vi "user_events_practice.vi"() -> ()   [LabVIEW 2020]
panel:
  out "all upper case string":string
  in  "Change to Upper":cluster{"string":string}={"string"="exaMple"}
  in  "stop":bool
  out "error out":errorcluster
  out "Type":u32
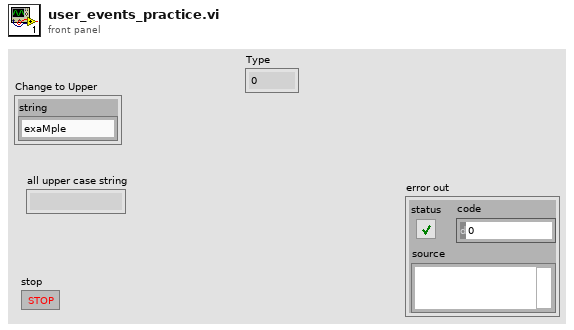
[diagram p1: front panel]
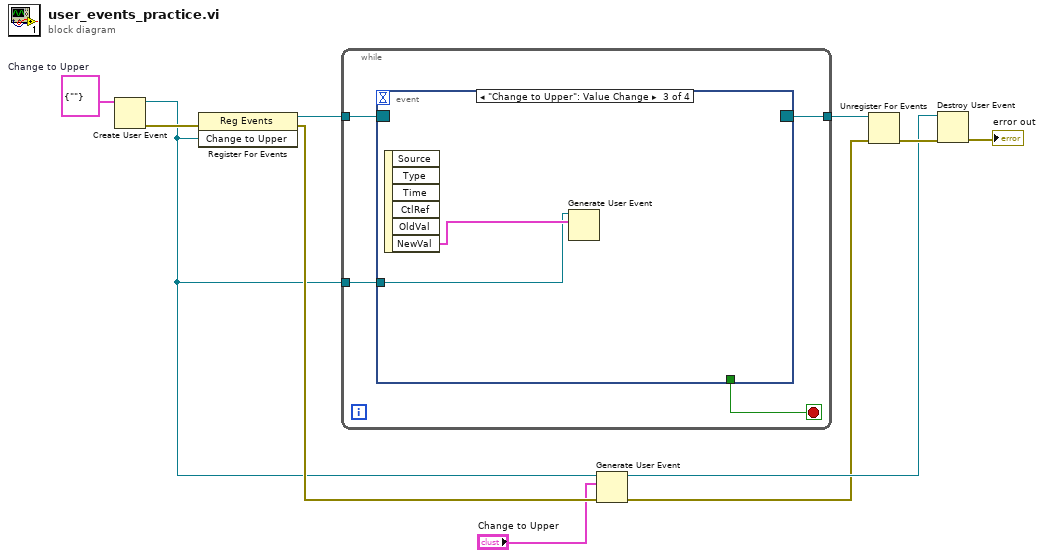
[diagram p0: block diagram]
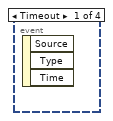
[diagram p2: hidden frame]
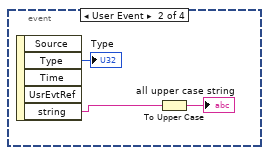
[diagram p3: hidden frame]
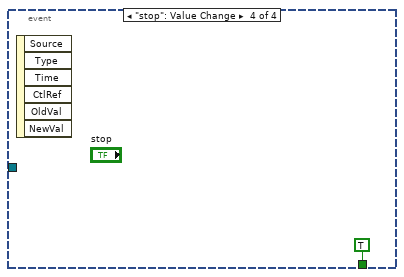
[diagram p4: hidden frame]
diagram:
  w11 = cluster{"string":string} {"string"=""}  # Change to Upper
  n1 = Create User Event(user event datatype=w11) -> (user event=w2:refnum<user-event>, error out=w10:errorcluster)  [unwired: 1 in]
  n2 = register-events(error in=w10, w2) -> (reference out=w9:refnum<event-registration>, error out=w7:errorcluster)  [unwired: 1 in]
  n3 = while {
    tunnel: w9 -> [w15]
    tunnel: [w14] -> w8
    tunnel: w2 -> [w12]
    stop <- w13 stop-if-true
    n4 = event shown="[2] \"Change to Upper\": Value Change" {
      selector: w15 -> [_ _ _ _]
      dyn-events: [_ _ _ _] -> w14
      timeout: _ -> [_ _ _ _]
      tunnel: [_ _ _ TRUE ("stop")] -> w13
      tunnel: w12 -> [_ _ w19 _]
      event Timeout {
        n5 = event-data() -> ()  [unwired: 1 in, 3 out]
      }
      event User Event {
        n6 = event-data() -> ("Type"=→"Type":u32, "string"=w17:string)  [unwired: 1 in, 3 out]
        n7 = To Upper Case(1:w17) -> (0:→"all upper case string":string)
      }
      event "Change to Upper": Value Change {
        n8 = event-data() -> ("NewVal"=w20:cluster{"string":string})  [unwired: 1 in, 5 out]
        n9 = Generate User Event(user event=w19, event data cluster=w20) -> ()  [unwired: 2 in, 2 out]
      }
      event "stop": Value Change {
        n10 = event-data() -> ()  [unwired: 1 in, 6 out]
      }
    }
  }
  n11 = Generate User Event(user event=w2, event data cluster="Change to Upper", error in=w7) -> (user event out=w3:refnum<user-event>, error out=w1:errorcluster)  [unwired: 1 in]
  n12 = Unregister For Events(event registration refnum=w8, error in=w1) -> (error out=w4:errorcluster)
  n13 = Destroy User Event(user event=w3, error in=w4) -> (error out=→"error out":errorcluster)
